vi "Zero if NaN.vi"(11 "Numeric":dbl) -> (3 "Numeric":dbl)   [LabVIEW 2021, in "RocketPlot.lvlib"]
uses:
  RocketPlot.lvlib
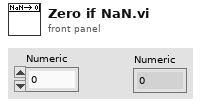
[diagram p1: front panel]
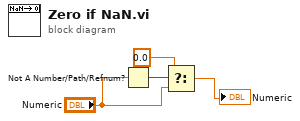
[diagram p0: block diagram]
diagram:
  n1 = Not A Number/Path/Refnum?(number/path/refnum="Numeric") -> (NaN/Path/Refnum?=w4:bool)
  n2 = Select(t=0.0, s=w4, f="Numeric") -> (s? t:f=→"Numeric":dbl)
